vi "WiringPi_Setup.vi"(8 "error in (no error)":errorcluster) -> (0 "error out":errorcluster)   [LabVIEW 2014, in "QwaveSys RPi Training Library.lvlib"]
uses:
  <vilib>/Q-Wave Systems/QwaveSys RPi Training Package (Demo)/Addons/QwaveSys RPi Training Library.lvlib
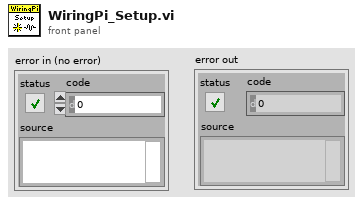
[diagram p1: front panel]
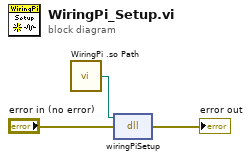
[diagram p0: block diagram]
diagram:
  n1 = call <vilib>:"WiringPi .so Path.vi"() -> ("WiringPi .so Path"=w1:path)  [unwired: 5 in]
  n2 = dll-call lib="libwiringPi.so" fn="wiringPiSetup"(path in=w1, error in="error in (no error)") -> (error out=→"error out":errorcluster)  [unwired: 2 in, 1 out]
